vi "From String.vi"(8 "error in (no error)":errorcluster, 10 "data":string, 11 "csv-formatter Config in":refnum<class "csv-formatter Config.lvclass">) -> (0 "error out":errorcluster, 3 "csv-formatter Config out":refnum<class "csv-formatter Config.lvclass">)   [LabVIEW 2015, in "csv-formatter Config.lvclass"]
uses:
  csv-formatter Config.lvclass
  csv-formatter Config.lvclass/csv-formatter Config.ctl
  <vilib>/NI/Configuration Framework/serializable configuration/NISE_CEF_serializable configuration.lvclass
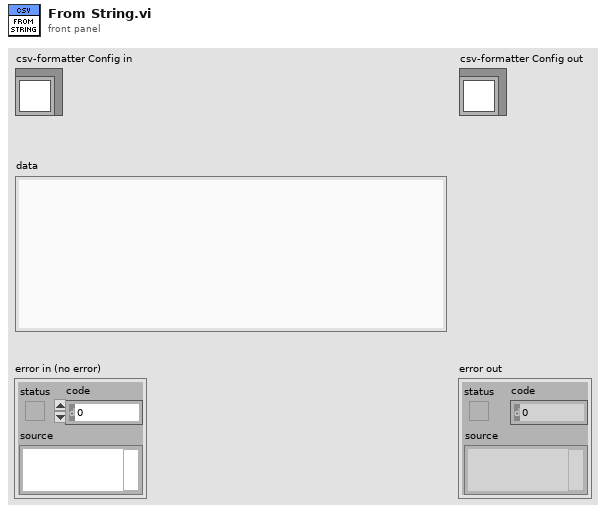
[diagram p1: front panel]
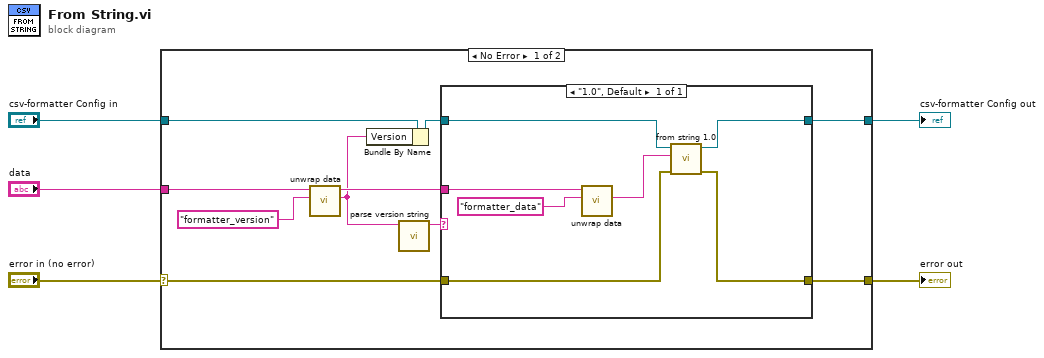
[diagram p0: block diagram]
diagram:
  n1 = case shown="No Error" "error in (no error)" {
    selector: "error in (no error)" -> [w14 w24]
    tunnel: [w13 w24] -> w5
    tunnel: [w12 w23] -> w1
    tunnel: "csv-formatter Config in" -> [w15 w23]
    tunnel: "data" -> [w10 _]
    frame No Error {
      n2 = call <vilib>:"unwrap data.vi"("identifier"="formatter_version", "data to unwrap"=w10) -> ("unwrapped data"=w6:string, "remaining string"=w9:string)  [unwired: 8 in]
      n3 = Bundle By Name(cluster=w15, "Version"=w6) -> (w7:refnum<class "csv-formatter Config.lvclass">)
      n4 = call <vilib>:"parse version string.vi"("full version"=w6) -> ("major.minor version"=w11:string)  [unwired: 7 in, 3 out]
      n5 = case shown="\"1.0\", Default" w11 {
        tunnel: w7 -> [w17]
        tunnel: w9 -> [w21]
        tunnel: w14 -> [w19]
        tunnel: [w18] -> w13
        tunnel: [w16] -> w12
        frame "1.0", Default {
          n6 = call <vilib>:"unwrap data.vi"("identifier"="formatter_data", "data to unwrap"=w21) -> ("unwrapped data"=w20:string)  [unwired: 8 in, 1 out]
          n7 = call-dynamic "from string 1.0.vi"("error in (no error)"=w19, "data"=w20, "Formatter Config in"=w17) -> ("error out"=w18:errorcluster, "Formatter Config out"=w16:refnum<class "csv-formatter Config.lvclass">)  [unwired: 7 in]
        }
      }
    }
    frame Error {
    }
  }
  "error out" <- w5
  "csv-formatter Config out" <- w1
